vi "Target Read Motor Sensors.vi"(8 "Error In":errorcluster, 11 "Motion Handle":refnum<k21>="nism://NI-PXIe8880-2F1836AB/AKM74L Motor") -> (0 "Error Out":errorcluster, 3 "Motor Sensors":T1)   [LabVIEW 2018, in "COBRA Kollmorgen Motor IO Library.lvlib"]
uses:
  COBRA Kollmorgen Motor IO Library.lvlib
  Target Motor Sensors.ctl
  <resource>/objmgr/nimcai.rc
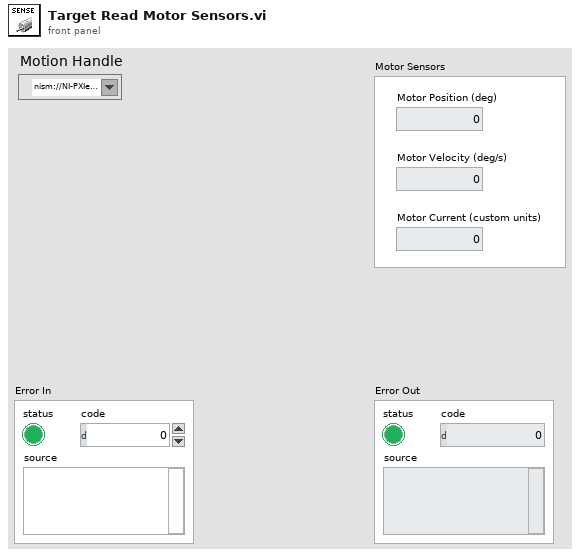
[diagram p1: front panel]
types:
  T1 = typedef "COBRA Kollmorgen Motor IO Library.lvlib/Target Motor Sensors.ctl" = cluster{"Motor Position (deg)":dbl, "Motor Velocity (deg/s)":dbl, "Motor Current (custom units)":dbl}
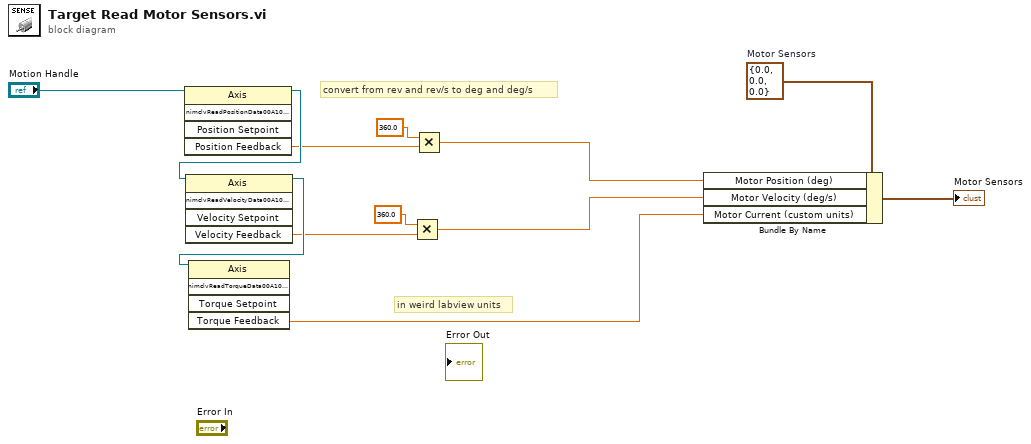
[diagram p0: block diagram]
diagram:
  w2 = T1 {"Motor Position (deg)"=0.0, "Motor Velocity (deg/s)"=0.0, "Motor Current (custom units)"=0.0}  # Motor Sensors
  # "in weird labview units"
  # "convert from rev and rev/s to deg and deg/s"
  n1 = invoke class="Axis" method="nimclvReadPositionData00A10001"(reference="Motion Handle") -> (reference out=w12:refnum<k21>, "Position Feedback"=w10:dbl)  [unwired: 4 in, 3 out]
  n2 = invoke class="Axis" method="nimclvReadVelocityData00A10001"(reference=w12) -> (reference out=w11:refnum<k21>, "Velocity Feedback"=w7:dbl)  [unwired: 4 in, 3 out]
  n3 = invoke class="Axis" method="nimclvReadTorqueData00A10001"(reference=w11) -> ("Torque Feedback"=w3:dbl)  [unwired: 4 in, 4 out]
  n4 = Multiply(x=360.0, y=w7) -> (x*y=w4:dbl)
  n5 = Multiply(x=360.0, y=w10) -> (x*y=w5:dbl)
  n6 = Bundle By Name(cluster=w2, "Motor Position (deg)"=w5, "Motor Velocity (deg/s)"=w4, "Motor Current (custom units)"=w3) -> (→"Motor Sensors":T1)
